vi "DAQmx.44xx.Get Fs Min and Max.vi"(8 "error in (no error)":errorcluster, 11 "DAQmx Device Name":tag) -> (0 "error out":errorcluster, 1 "Fs Min":dbl, 2 "Fs Max":dbl)   [LabVIEW 2019, in "DAQmx.lvclass"]
uses:
  DAQmx.lvclass
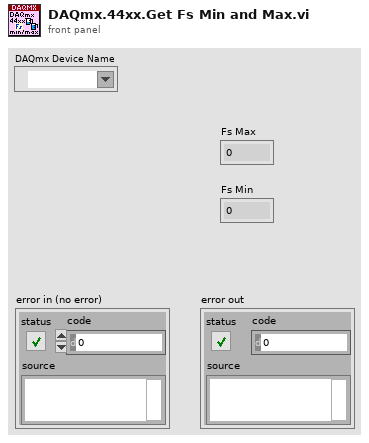
[diagram p1: front panel]
types:
  T1 = typedef "DAQmx.lvclass/DAQ.Config.Device Type--enum.ctl" = enum16{"None", "USB-4431", "PXI-446x"}
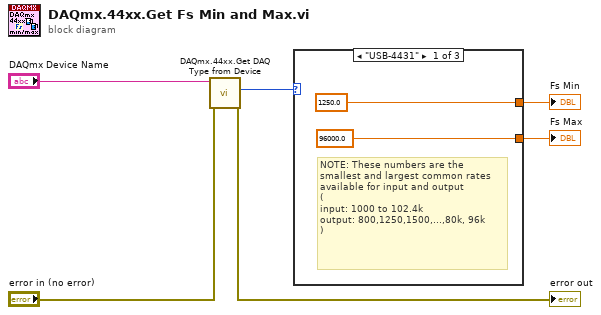
[diagram p0: block diagram]
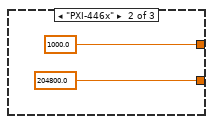
[diagram p2: hidden frame]
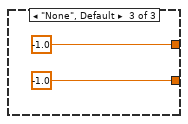
[diagram p3: hidden frame]
diagram:
  n1 = call "DAQmx.44xx.Get DAQ Type from Device.vi"("error in (no error)"="error in (no error)", "DAQmx Device Name"="DAQmx Device Name") -> ("error out"=→"error out":errorcluster, "DAQ Type"=w4:T1)  [unwired: 7 in, 1 out]
  n2 = case shown="\"USB-4431\"" w4 {
    tunnel: [1250.0 1000.0 -1.0] -> w6
    tunnel: [96000.0 ("AI.Min") 204800.0 ("AI.Min") -1.0 ("AI.Min")] -> w5
    frame "USB-4431" {
      # "NOTE: These numbers are the smallest and largest common rates available for input and output\n(\ninput: 1000 to 102.4k\noutput: 800,1250,1500,...,80k, 96k\n)"
    }
    frame "PXI-446x" {
    }
    frame "None", Default {
    }
  }
  "Fs Min" <- w6
  "Fs Max" <- w5
